vi "ex10-1.vi"() -> ()   [LabVIEW 2013]
uses:
  <vilib>/NXT/Block Support/NXT_InputPort.ctl
  <vilib>/NXT/Block Support/NXT_OutputPort.ctl
  <vilib>/NXT/Dual Mode Library/Sensors/EV3_Color_Reflect.vi
  <vilib>/NXT/NXTIO Xnodes/NXTIONodeSubVIs/NXTMoveMotors.vi
  <vilib>/NXT/NXTIO Xnodes/AddressXNode/NXTIOAddress.xnode
  <vilib>/NXT/NXTIO Xnodes/NXTIOXNode/NXTIO.xnode
  <vilib>/NXT/Subs/LVHSConnector.ctl
  <vilib>/NXT/LegoClasses/BrickReference/BrickReference.lvclass
panel:
  out "Waveform Graph":dbl[][](graph)
  out "left":dbl[][](array[numeric])
  in  "stop 2":bool
  # "left               right"
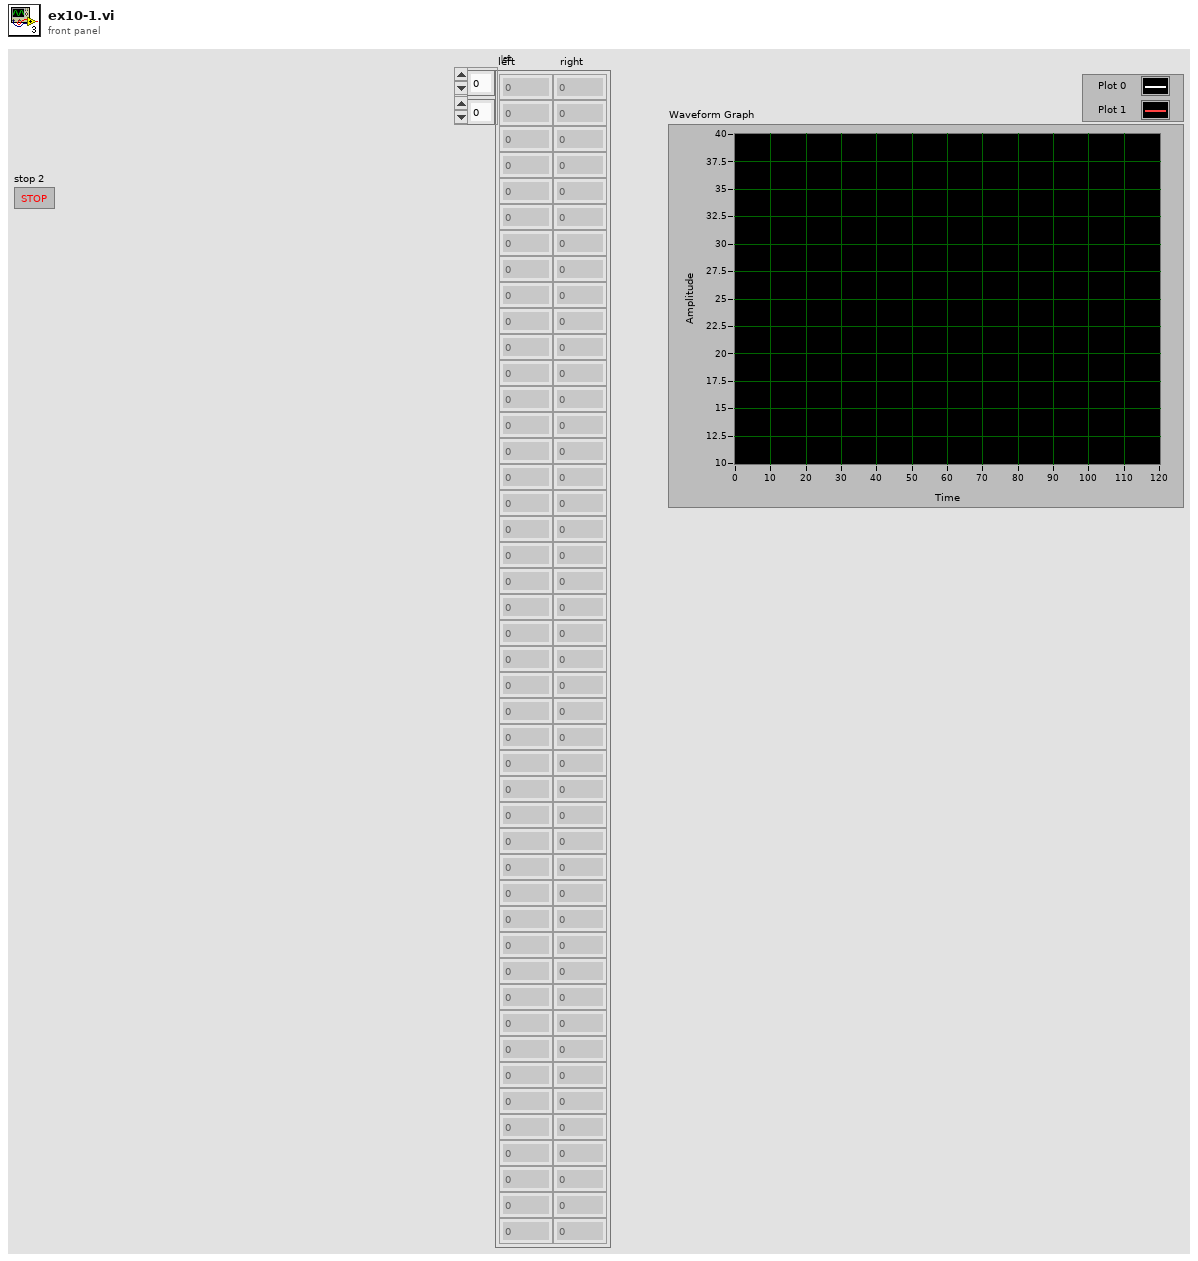
[diagram p1: front panel]
types:
  T1 = typedef "NXT_InputPort.ctl" = u32
  T2 = typedef "LVHSConnector.ctl" = refnum<class "BrickReference.lvclass">
  T3 = typedef "NXT_OutputPort.ctl" = u8
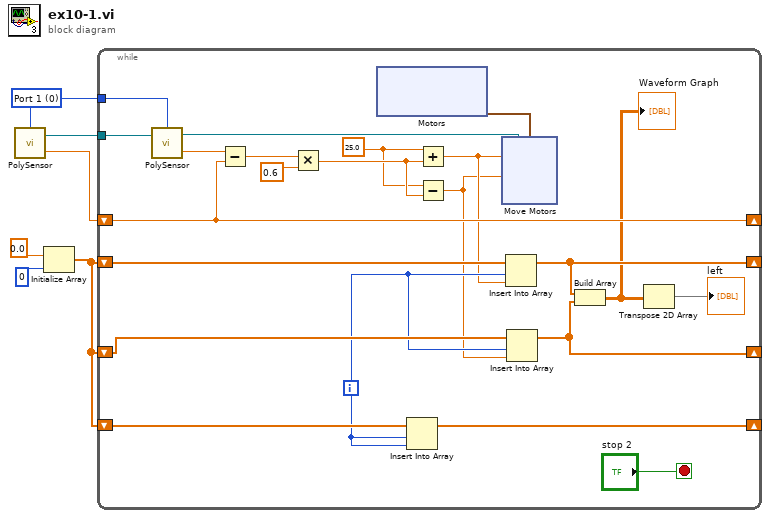
[diagram p0: block diagram]
diagram:
  w5 = T1 0 items=["Port 1", "Port 2", "Port 3", "Port 4"] ("Port (Port 1)")
  n1 = call-poly <vilib>:"PolySensor.vi"("Port (Port 1)"=w5) -> ("Scaled Value"=w6:sgl, "NXT/EV3"=w4:T2)  [unwired: 2 in]
  n2 = Initialize Array(0.0 ("element"), 0 ("dimension size")) -> (w1:dbl[])
  n3 = while {
    shift-right: [w22] -> _
    shift-left: w6 -> [w22]
    tunnel: w5 -> [w25]
    tunnel: w4 -> [w24]
    shift-right: [w13] -> _
    shift-left: w1 -> [w18]
    shift-right: [w12] -> _
    shift-left: w1 -> [w17]
    shift-right: [w14] -> _
    shift-left: w1 -> [w15]
    i -> [w10]
    stop <- "stop 2" stop-if-true
    w20 = 25.0 ("y")
    n4 = call-poly <vilib>:"PolySensor.vi"("NXT/EV3"=w24, "Port (Port 1)"=w25) -> ("Scaled Value"=w23:sgl, "NXT/EV3"=w19:T2)  [unwired: 1 in]
    n5 = Subtract(x=w23, y=w22) -> (x-y=w28:sgl)
    n6 = Multiply(x=w28, y=0.6) -> (x*y=w21:dbl)
    n7 = xnode "Motors"() -> ("Motor"=w27:cluster{"Port":T3, "Port":T3})
    n8 = Insert Into Array(array=w15, index=w10, new element=w10) -> (w14:dbl[])
    n9 = Add(x=w20, y=w21) -> (x+y=w9:dbl)
    n10 = Subtract(x=w20, y=w21) -> (x-y=w8:dbl)
    n11 = xnode "Move Motors"("Power/Speed 2"=w8, "Power/Speed 1"=w9, "Motors"=w27, "NXT/EV3"=w19) -> ()  [unwired: 1 out]
    n12 = Insert Into Array(array=w18, index=w10, new element=w9) -> (w13:dbl[])
    n13 = Insert Into Array(array=w17, index=w10, new element=w8) -> (w12:dbl[])
    n14 = Build Array(w13, w12) -> (w7:dbl[][])
    "Waveform Graph" <- w7
    n15 = Transpose 2D Array(2D array=w7) -> (transposed array=→"left":dbl[][])
  }
